vi "SW_BoolArryToNumber.vi"(0 "L1":bool[](array[boolean]), 1 "L 2":bool[](array[boolean]), 2 "L 3":bool[](array[boolean]), 3 "L 4":bool[](array[boolean]), 4 "L 5":bool[](array[boolean]), 5 "L 6":bool[](array[boolean]), 6 "L 7":bool[](array[boolean]), 7 "L 8":bool[](array[boolean])) -> (20 "H":string, 21 "L":string)   [LabVIEW 2018]
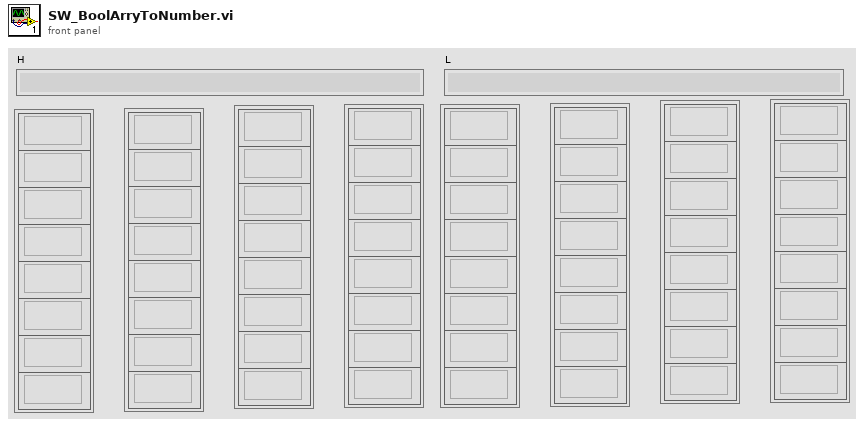
[diagram p1: front panel]
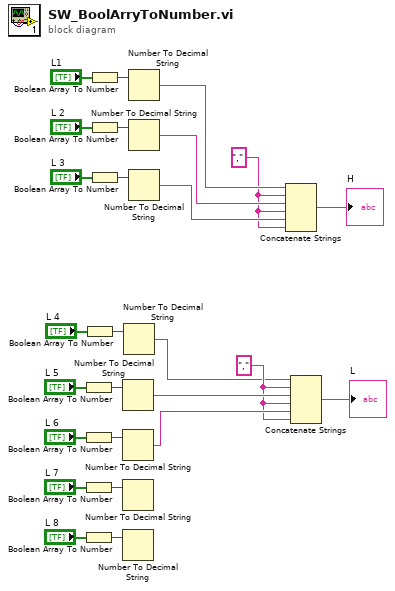
[diagram p0: block diagram]
diagram:
  w2 = ","
  w7 = ","
  n1 = Boolean Array To Number(Boolean array="L 5") -> (number=w21:u32)
  n2 = Boolean Array To Number(Boolean array="L 6") -> (number=w20:u32)
  n3 = Boolean Array To Number(Boolean array="L 7") -> (number=w19:u32)
  n4 = Boolean Array To Number(Boolean array="L 8") -> (number=w18:u32)
  n5 = Boolean Array To Number(Boolean array="L 4") -> (number=w22:u32)
  n6 = Boolean Array To Number(Boolean array="L1") -> (number=w26:u32)
  n7 = Boolean Array To Number(Boolean array="L 2") -> (number=w24:u32)
  n8 = Boolean Array To Number(Boolean array="L 3") -> (number=w23:u32)
  n9 = Number To Decimal String(number=w21) -> (decimal integer string=w4:string)  [unwired: 1 out]
  n10 = Number To Decimal String(number=w20) -> (decimal integer string=w3:string)  [unwired: 1 out]
  n11 = Number To Decimal String(number=w19) -> ()  [unwired: 2 out]
  n12 = Number To Decimal String(number=w18) -> ()  [unwired: 2 out]
  n13 = Number To Decimal String(number=w22) -> (decimal integer string=w1:string)  [unwired: 1 out]
  n14 = Number To Decimal String(number=w26) -> (decimal integer string=w10:string)  [unwired: 1 out]
  n15 = Number To Decimal String(number=w24) -> (decimal integer string=w9:string)  [unwired: 1 out]
  n16 = Number To Decimal String(number=w23) -> (decimal integer string=w8:string)  [unwired: 1 out]
  n17 = Concatenate Strings(w10, w7, w9, w7, w8, w7) -> (→"H":string)
  n18 = Concatenate Strings(w1, w2, w4, w2, w3, w2) -> (→"L":string)
